vi "UTIL_Round.vi"(10 "Significant decimal":dbl, 11 "Number":dbl) -> (3 "Numeric":dbl)   [LabVIEW 2024]
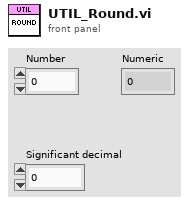
[diagram p1: front panel]
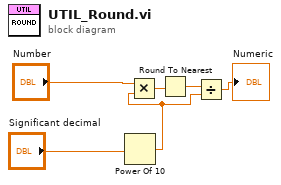
[diagram p0: block diagram]
diagram:
  n1 = Power Of 10(x="Significant decimal") -> (10^x=w1:dbl)
  n2 = Multiply(x="Number", y=w1) -> (x*y=w4:dbl)
  n3 = Round To Nearest(number=w4) -> (nearest integer value=w5:dbl)
  n4 = Divide(x=w5, y=w1) -> (x/y=→"Numeric":dbl)
